vi "Header Footer Transform Header Footer [ ].vi"(7 "Header or Footer [ ]":T15, 11 "error in (no error)":errorcluster) -> (8 "Header or Footer Complete Cluster":T1, 15 "error out":errorcluster)   [LabVIEW 2019]
doc: "Version 1.0\nDeveloped by Jean-Marc Simard\nCopyright © 2010, Exaprom Inc.\nAll rights reserved.\nLicense: BSD\n\nWith iTextSharp 4.1.6 (http://itextsharp.sourceforge.net)\nunder Mozilla Public License Version 1.1\n(http://www.mozilla.org/MPL/MPL-1.1.html)"
uses:
  <userlib>/Exaprom PDF/LV Class/Header and Footer Class/VIs/Controls/Header Footer [ ] V2.ctl
  <userlib>/Exaprom PDF/LV Class/Header and Footer Class/VIs/Controls/Header Footer cluster V2.ctl
  <userlib>/Exaprom PDF/Controls/Header, Footer and Watermark Controls/Header or Footer.ctl
  <userlib>/Exaprom PDF/Controls/Header, Footer and Watermark Controls/Header Footer Type.ctl
  <userlib>/Exaprom PDF/Controls/Header, Footer and Watermark Controls/Header footer horiz alignment.ctl
  <userlib>/Exaprom PDF/Controls/Table Controls/Cell Vertical alignment.ctl
  <userlib>/Exaprom PDF/Controls/Text Controls/Line spacing.ctl
  <userlib>/Exaprom PDF/Controls/Header, Footer and Watermark Controls/Page number.ctl
  <userlib>/Exaprom PDF/Controls/Font Controls/Font complete cluster horizontal.ctl
  <userlib>/Exaprom PDF/Controls/Font Controls/Font size.ctl
  <userlib>/Exaprom PDF/Controls/Font Controls/Font color.ctl
  <userlib>/Exaprom PDF/Controls/Font Controls/Type and encoding.ctl
  <userlib>/Exaprom PDF/Controls/Text Controls/Unicode/Type and run direction.ctl
  C:/Program Files/National Instruments/LabVIEW 2019/user.lib/Exaprom PDF/DLL/itextsharp.dll
  DLL/itextsharp.dll
  <userlib>/Exaprom PDF/Controls/Header, Footer and Watermark Controls/Header Footer Line.ctl
  <userlib>/Exaprom PDF/Controls/Header, Footer and Watermark Controls/Header Footer Complete Cluster.ctl
  <userlib>/Exaprom PDF/Controls/Header, Footer and Watermark Controls/Header or Footer Position.ctl
  <userlib>/Exaprom PDF/Controls/Header, Footer and Watermark Controls/Header Footer Cluster with references.ctl
  <userlib>/Exaprom PDF/Controls/Text Controls/Text type.ctl
panel:
  # "X"
  # "Y"
  # "X"
  # "Y"
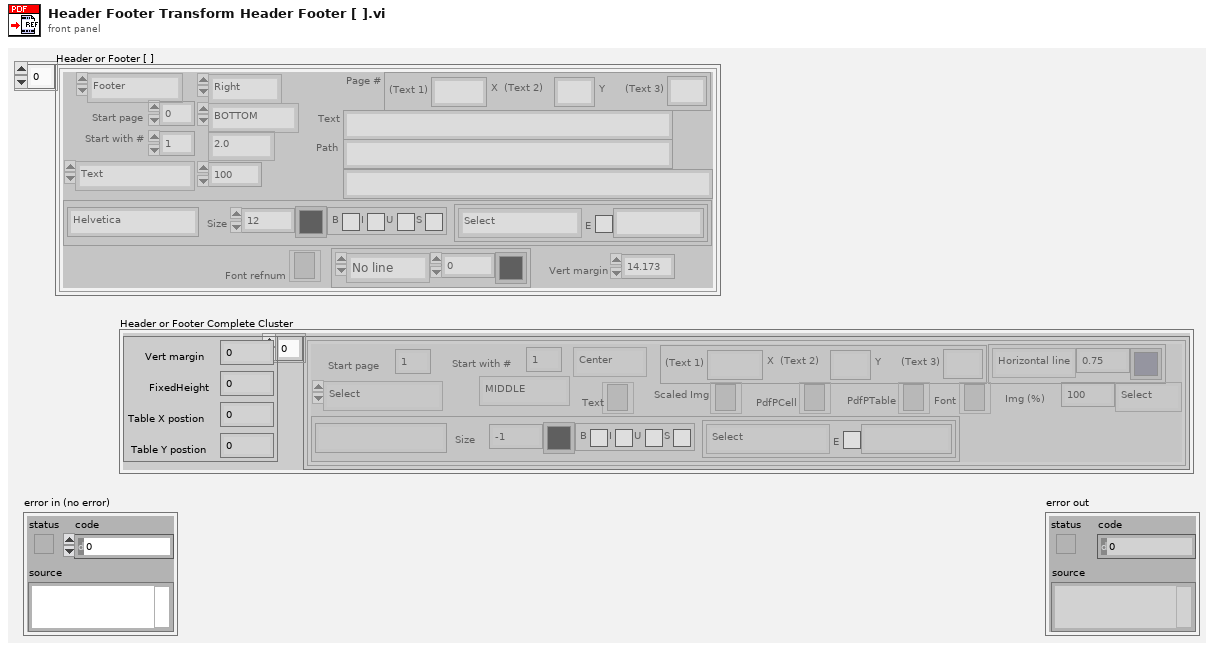
[diagram p1: front panel]
types:
  T1 = typedef "Header Footer Complete Cluster.ctl" = cluster{"Table position":T2, "Header Footer Cluster with references [ ]":T3[]}
  T2 = typedef "Header or Footer Position.ctl" = cluster{"Vert margin":dbl, "FixedHeight":dbl, "Table X postion":dbl, "Table Y postion":dbl}
  T3 = typedef "Header Footer Cluster with references.ctl" = cluster{"Start page":i32, "Type":T4, "Start with #":i32, "Alignment":T5, "Vertical Alignement":T6, "Page #":T7, "Text":refnum<k24>, "Scaled Img":refnum<k24>, "PdfPCell":refnum<k24>, "PdfPTable":refnum<k24>, "Font Cluster":T8, "Font ":refnum<k24>, "Img (%)":sgl, "Line":cluster{"Line":T13, "Thickness (points)":sgl, "Colour":T10}, "Line spacing":T14}
  T4 = typedef "Header Footer Type.ctl" = enum16{"Select", "Text", "Text + hyperlink", "Page number", "Image", "Image + hyperlink"}
  T5 = typedef "Header footer horiz alignment.ctl" = enum16{"Left", "Center", "Right"}
  T6 = typedef "Cell Vertical alignment.ctl" = enum16{"TOP", "MIDDLE", "BOTTOM"}
  T7 = typedef "Page number.ctl" = cluster{"Text 1":string, "Text 2":string, "Text 3":string}
  T8 = typedef "Font complete cluster horizontal.ctl" = cluster{"Name":string, "Size":T9, "Color":T10, "Style":cluster{"Bold":bool, "Italic":bool, "Underline":bool, "Strikeout":bool}, "Type":T11}
  T9 = typedef "Font size.ctl" = sgl
  T10 = typedef "Font color.ctl" = u32
  T11 = typedef "Type and encoding.ctl" = cluster{"Type&direction":T12, "Embedded":bool, "Encoding":string}
  T12 = typedef "Type and run direction.ctl" = enum16{"Select", "ASCII", "UTF-16", "UTF-16 (default)", "UTF-16 (LTR)", "UTF-16 (RTL)"}
  T13 = typedef "Header Footer Line.ctl" = enum16{"No line", "Horizontal line"}
  T14 = typedef "Line spacing.ctl" = enum16{"Select", "1.0", "1.5", "2.0"}
  T15 = typedef "Header Footer [ ] V2.ctl" = T16[]
  T16 = typedef "Header Footer cluster V2.ctl" = cluster{"Header or Footer":T17, "Start page":i32, "Start with #":i32, "Type":T4, "Alignment":T5, "Vertical Alignement":T6, "Line spacing":T14, "Image (%)":sgl, "Page #":T7, "Text":string, "Path":string, "Font":T8, "Font refnum":refnum<k24>, "Line":cluster{"Line":T13, "Thickness (points)":sgl, "Colour":T10}, "Vert margin":dbl, "Hyperlink":string}
  T17 = typedef "Header or Footer.ctl" = enum16{"Header", "Footer"}
  T18 = typedef "Text type.ctl" = enum16{"empty", "Text", "Hyperlink"}
  T19 = cluster{"Text type":T18, "Text":string, "Hyperlink":string}[]
  T20 = cluster{"Text type":T18, "Text":string, "Hyperlink":string}
  T21 = cluster{"Line":T13, "Thickness (points)":sgl, "Colour":T10}
  T22 = cluster{"Table position":T2, "Header Footer Cluster with references [ ]":T3[]}
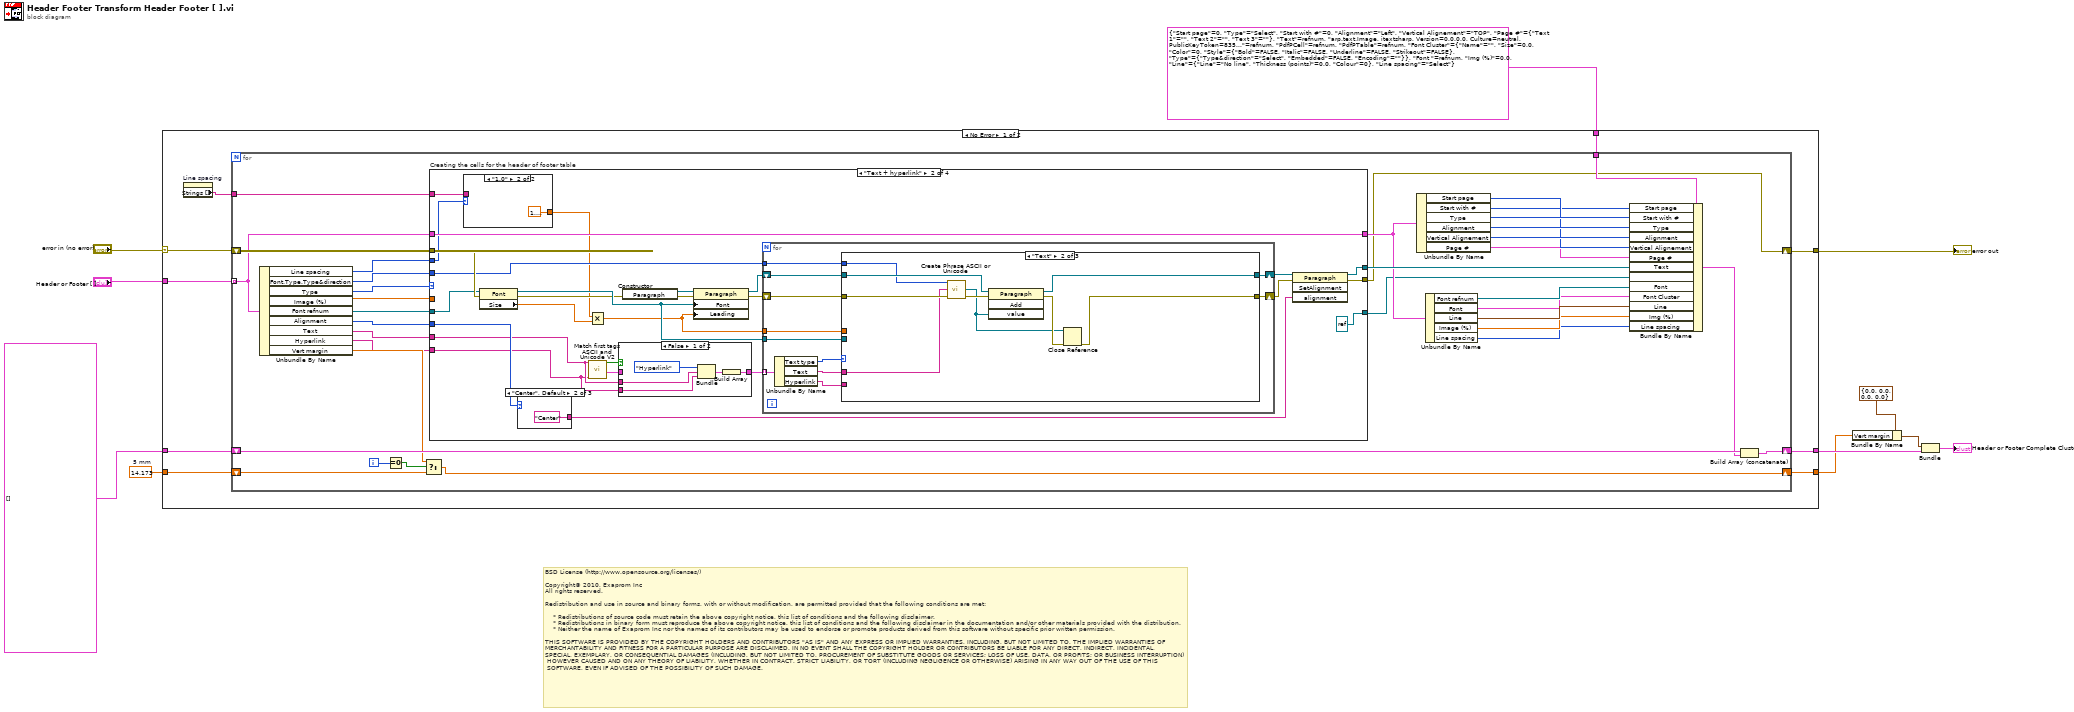
[diagram p0: block diagram]
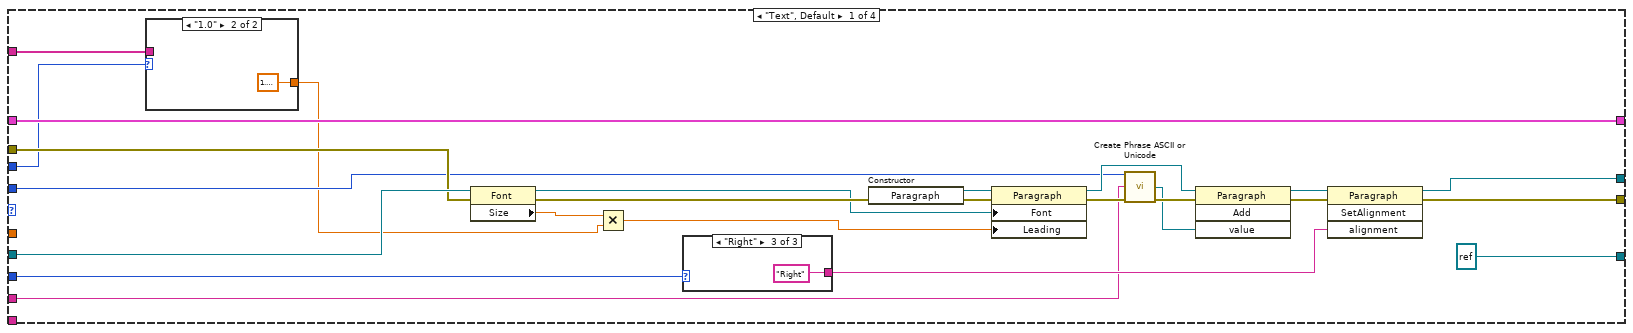
[diagram p2: hidden frame]
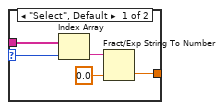
[diagram p3: hidden frame]
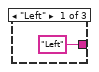
[diagram p4: hidden frame]
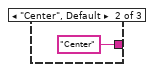
[diagram p5: hidden frame]
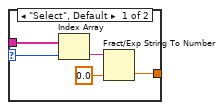
[diagram p6: hidden frame]
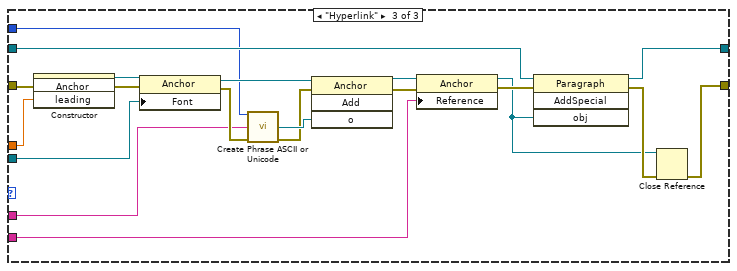
[diagram p9: hidden frame]
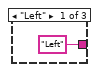
[diagram p10: hidden frame]
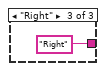
[diagram p11: hidden frame]
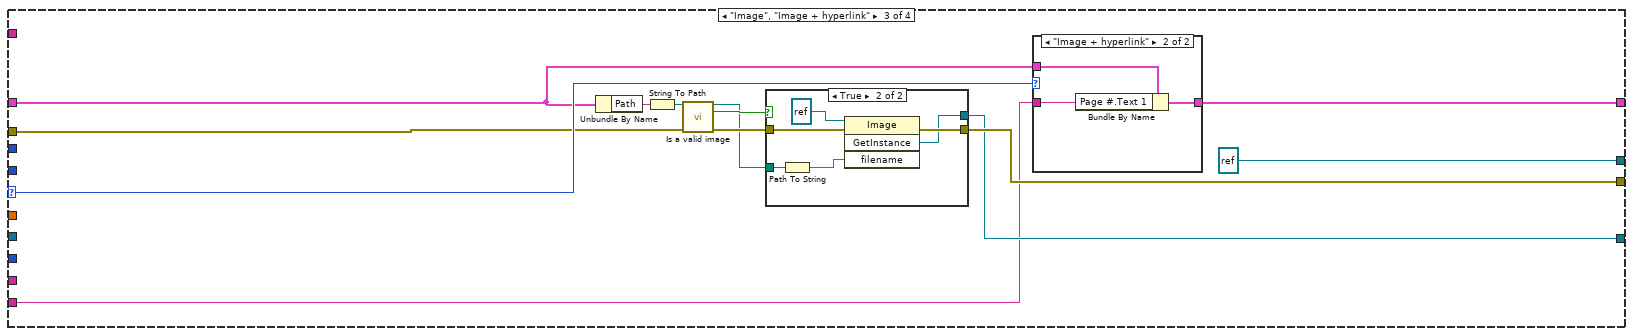
[diagram p12: hidden frame]
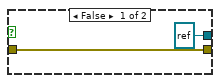
[diagram p13: hidden frame]
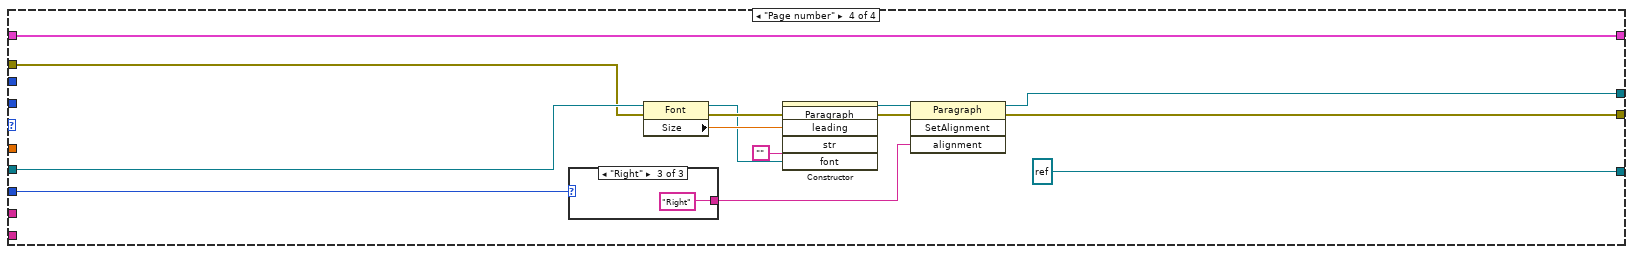
[diagram p15: hidden frame]
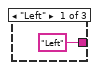
[diagram p16: hidden frame]
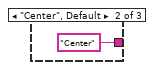
[diagram p17: hidden frame]
diagram:
  w5 = 14.173  # 5 mm
  # "BSD License (http://www.opensource.org/licenses/)\n\nCopyright© 2010, Exaprom Inc\nAll rights reserved.\n\nRedistribution and use in source and binary forms, with or without modification, are permitted provided that the following conditions are met:\n\n    * Redistributions of source code must retain the above copyright notice, this list of conditions and the following disclaimer.\n    * Redistributions in binary form must reproduce the above copyright notice, this list of conditions and the following disclaimer in the documentation and/or other materials provided with the distribution.\n    * Neither the name of Exaprom Inc nor the names of its contributors may be used to endorse or promote products derived from this software without specific prior written permission.\n\nTHIS SOFTWARE IS PROVIDED BY THE COPYRIGHT HOLDERS AND CONTRIBUTORS \"AS IS\" AND ANY EXPRESS OR IMPLIED WARRANTIES, INCLUDING, BUT NOT LIMITED TO, THE IMPLIED WARRANTIES OF \nMERCHANTABILITY AND FITNESS FOR A PARTICULAR PURPOSE ARE DISCLAIMED. IN NO EVENT SHALL THE COPYRIGHT HOLDER OR CONTRIBUTORS BE LIABLE FOR ANY DIRECT, INDIRECT, INCIDENTAL,\nSPECIAL, EXEMPLARY, OR CONSEQUENTIAL DAMAGES (INCLUDING, BUT NOT LIMITED TO, PROCUREMENT OF SUBSTITUTE GOODS OR SERVICES; LOSS OF USE, DATA, OR PROFITS; OR BUSINESS INTERRUPTION)\n HOWEVER CAUSED AND ON ANY THEORY OF LIABILITY, WHETHER IN CONTRACT, STRICT LIABILITY, OR TORT (INCLUDING NEGLIGENCE OR OTHERWISE) ARISING IN ANY WAY OUT OF THE USE OF THIS\n SOFTWARE, EVEN IF ADVISED OF THE POSSIBILITY OF SUCH DAMAGE."
  n1 = case shown="No Error" "error in (no error)" {
    selector: "error in (no error)" -> [w16 w218]
    tunnel: "Header or Footer [ ]" -> [w15 _]
    tunnel: [w20 w218] -> w11
    tunnel: T3 {"Start page"=0, "Type"=enum."Select", "Start with #"=0, "Alignment"=enum."Left", "Vertical Alignement"=enum."TOP", "Page #"={"Text 1"="", "Text 2"="", "Text 3"=""}, "Text"=refnum, "Scaled Img"=refnum, "PdfPCell"=refnum, "PdfPTable"=refnum, "Font Cluster"={"Name"="", "Size"=0.0, "Color"=0, "Style"={"Bold"=FALSE, "Italic"=FALSE, "Underline"=FALSE, "Strikeout"=FALSE}, "Type"={"Type&direction"=enum."Select", "Embedded"=FALSE, "Encoding"=""}}, "Font "=refnum, "Img (%)"=0.0, "Line"={"Line"=enum."No line", "Thickness (points)"=0.0, "Colour"=0}, "Line spacing"=enum."Select"} ("Header Footer Cluster with references") -> [w19 _]
    tunnel: T3[] [] ("Header Footer Cluster with references [ ]") -> [w18 w217]
    tunnel: [w17 w217] -> w7
    tunnel: [w14 w216] -> w2
    tunnel: w5 -> [w13 w216]
    frame No Error {
      n2 = property on="Line spacing" class="Enum (strict)"() -> ("Strings []"=w12:string[])  [unwired: 2 in, 2 out]
      n3 = for {
        tunnel: w15 -> [w41] mode=indexing
        tunnel: w19 -> [w50]
        shift-right: [w43] -> w17
        shift-left: w18 -> [w42]
        shift-right: [w36] -> w20
        shift-left: w16 -> [w39]
        shift-right: [w29] -> w14
        shift-left: w13 -> [w30]
        tunnel: w12 -> [w22]
        i -> [w32]
        n4 = Unbundle By Name(w41) -> ("Line spacing"=w23:T14, "Font.Type.Type&direction"=w27:T12, "Type"=w52:T4, "Image (%)"=w53:sgl, "Font refnum"=w55:refnum<k24>, "Alignment"=w54:T5, "Text"=w51:string, "Hyperlink"=w25:string, "Vert margin"=w26:dbl)
        n5 = Equal To 0?(x=w32) -> (x = 0?=w31:bool)
        n6 = Select(t=w26, s=w31, f=w30) -> (s? t:f=w29:dbl)
        n7 = case "Creating the cells for the header of footer table" shown="\"Text + hyperlink\"" w52 {
          selector: w52 -> [_ _ w184 _]
          tunnel: w41 -> [w75 w113 w179 w207]
          tunnel: w55 -> [w80 w98 _ w212]
          tunnel: w54 -> [w79 w116 _ w211]
          tunnel: w53 -> [_ _ _ _]
          tunnel: w51 -> [w62 w101 _ _]
          tunnel: w39 -> [w78 w99 w176 w210]
          tunnel: [w73 w111 refnum<k24> refnum ("new reference") w206] -> w44
          tunnel: [refnum<k24> refnum ("GetInstanceImage OUT") refnum<k24> refnum ("GetInstanceImage OUT") w182 refnum<k24> refnum ("GetInstanceImage OUT")] -> w38
          tunnel: [w77 w114 w185 w209] -> w36
          tunnel: [w75 w113 w183 w207] -> w40
          tunnel: w27 -> [w61 w97 _ _]
          tunnel: w25 -> [_ w100 w174 _]
          tunnel: w23 -> [w56 w91 _ _]
          tunnel: w22 -> [w59 w92 _ _]
          frame "Text", Default {
            n8 = case shown="\"1.0\"" w56 {
              selector: w56 -> [w81 _]
              tunnel: w59 -> [w83 _]
              tunnel: [w82 sgl 1.1] -> w57
              frame "Select", Default {
                n9 = Index Array(array=w83, index=w81) -> (element=w85:string)
                n10 = Fract/Exp String To Number(string=w85, default (0 dbl)=sgl 0.0 ("default (0 DBL)")) -> (number=w82:sgl)  [unwired: 3 out]
              }
              frame "1.0" {
              }
            }
            n11 = property class="Font"(reference=w80, error in=w78) -> (reference out=w69:refnum<k24>, error out=w72:errorcluster, "Size"=w68:sgl)
            n12 = Multiply(x=w68, y=w57) -> (x*y=w58:sgl)
            n13 = case shown="\"Right\"" w79 {
              tunnel: ["Left" "Center" "Right"] -> w74
              frame "Left" {
              }
              frame "Center", Default {
              }
              frame "Right" {
              }
            }
            n14 = constructor class="Paragraph"(error in=w72) -> (reference out=w70:refnum<k24>, error out=w71:errorcluster)  [unwired: 2 in, 1 out]
            n15 = property class="Paragraph"(reference=w70, error in=w71, "Font"=w69, "Leading"=w58) -> (reference out=w65:refnum<k24>, error out=w64:errorcluster)
            n16 = call <userlib>:"Create Phrase ASCII or Unicode.vi"("Character type"=w61, "Text"=w62, "error in (no error)"=w64) -> ("Phrase refnum"=w60:refnum<k24>, "error out"=w63:errorcluster)  [unwired: 10 in, 1 out]
            n17 = invoke class="Paragraph" method="Add"(reference=w65, error in=w63, "value"=w60) -> (reference out=w67:refnum<k24>, error out=w66:errorcluster)  [unwired: 1 in, 2 out]
            n18 = invoke class="Paragraph" method="SetAlignment"(reference=w67, error in=w66, "alignment"=w74) -> (reference out=w73:refnum<k24>, error out=w77:errorcluster)  [unwired: 1 in, 2 out]
          }
          frame "Text + hyperlink" {
            n19 = case shown="\"1.0\"" w91 {
              selector: w91 -> [w117 _]
              tunnel: w92 -> [w119 _]
              tunnel: [w118 sgl 1.1] -> w90
              frame "Select", Default {
                n20 = Index Array(array=w119, index=w117) -> (element=w121:string)
                n21 = Fract/Exp String To Number(string=w121, default (0 dbl)=sgl 0.0 ("default (0 DBL)")) -> (number=w118:sgl)  [unwired: 3 out]
              }
              frame "1.0" {
              }
            }
            n22 = property class="Font"(reference=w98, error in=w99) -> (reference out=w110:refnum<k24>, error out=w105:errorcluster, "Size"=w109:sgl)
            n23 = case shown="\"Center\", Default" w116 {
              tunnel: ["Left" "Center" "Right"] -> w112
              frame "Left" {
              }
              frame "Center", Default {
              }
              frame "Right" {
              }
            }
            n24 = Multiply(x=w90, y=w109) -> (x*y=w93:sgl)
            n25 = call <userlib>:"Match first tags ASCII and Unicode V2.vi"("Hyperlink"=w100, "Text"=w101) -> ("Array"=w108:T19, "Find tag ?"=w106:bool)  [unwired: 3 in, 5 out]
            n26 = case shown="False" w106 {
              tunnel: [w123 w128] -> w107
              tunnel: w108 -> [_ w128]
              tunnel: w101 -> [w125 _]
              tunnel: w100 -> [w126 _]
              frame False {
                n27 = Bundle("Text type"=Text_type."Hyperlink", "Text"=w125, "Hyperlink"=w126) -> (w127:T20)  [unwired: 1 in]
                n28 = Build Array(w127) -> (w123:T19)
              }
              frame True {
              }
            }
            n29 = constructor class="Paragraph"(error in=w105) -> (reference out=w103:refnum<k24>, error out=w104:errorcluster)  [unwired: 2 in, 1 out]
            n30 = property class="Paragraph"(reference=w103, error in=w104, "Font"=w110, "Leading"=w93) -> (reference out=w94:refnum<k24>, error out=w102:errorcluster)
            n31 = for {
              shift-right: [w137] -> w95
              shift-left: w94 -> [w138]
              shift-right: [w136] -> w96
              shift-left: w102 -> [w139]
              tunnel: w107 -> [w135] mode=indexing
              tunnel: w93 -> [w131]
              tunnel: w110 -> [w130]
              tunnel: w97 -> [w129]
              n32 = Unbundle By Name(w135) -> ("Text type"=w134:T18, "Text"=w133:string, "Hyperlink"=w132:string)
              n33 = case shown="\"Text\"" w134 {
                tunnel: w139 -> [w141 w149 w164]
                tunnel: w138 -> [w140 w148 w159]
                tunnel: [w140 w147 w160] -> w137
                tunnel: [w141 w144 w155] -> w136
                tunnel: w133 -> [_ w146 w158]
                tunnel: w132 -> [_ _ w157]
                tunnel: w131 -> [_ _ w153]
                tunnel: w130 -> [_ _ w152]
                tunnel: w129 -> [_ w142 w151]
                frame "empty", Default {
                }
                frame "Text" {
                  n34 = call <userlib>:"Create Phrase ASCII or Unicode.vi"("Character type"=w142, "Text"=w146, "error in (no error)"=w149) -> ("Phrase refnum"=w143:refnum<k24>, "error out"=w150:errorcluster)  [unwired: 10 in, 1 out]
                  n35 = invoke class="Paragraph" method="Add"(reference=w148, error in=w150, "value"=w143) -> (reference out=w147:refnum<k24>, error out=w145:errorcluster)  [unwired: 1 in, 2 out]
                  n36 = Close Reference(reference=w143, error in (no error)=w145) -> (error out=w144:errorcluster)
                }
                frame "Hyperlink" {
                  n37 = constructor class="Anchor"(error in=w164, "leading"=w153) -> (reference out=w170:refnum<k24>, error out=w169:errorcluster)  [unwired: 2 in, 2 out]
                  n38 = property class="Anchor"(reference=w170, error in=w169, "Font"=w152) -> (reference out=w168:refnum<k24>, error out=w163:errorcluster)
                  n39 = call <userlib>:"Create Phrase ASCII or Unicode.vi"("Character type"=w151, "Text"=w158, "error in (no error)"=w163) -> ("Phrase refnum"=w165:refnum<k24>, "error out"=w162:errorcluster)  [unwired: 10 in, 1 out]
                  n40 = invoke class="Anchor" method="Add"(reference=w168, error in=w162, "o"=w165) -> (reference out=w166:refnum<k24>, error out=w167:errorcluster)  [unwired: 1 in, 2 out]
                  n41 = property class="Anchor"(reference=w166, error in=w167, "Reference"=w157) -> (reference out=w154:refnum<k24>, error out=w161:errorcluster)
                  n42 = invoke class="Paragraph" method="AddSpecial"(reference=w159, error in=w161, "obj"=w154) -> (reference out=w160:refnum<k24>, error out=w156:errorcluster)  [unwired: 1 in, 2 out]
                  n43 = Close Reference(reference=w154, error in (no error)=w156) -> (error out=w155:errorcluster)
                }
              }
            }
            n44 = invoke class="Paragraph" method="SetAlignment"(reference=w95, error in=w96, "alignment"=w112) -> (reference out=w111:refnum<k24>, error out=w114:errorcluster)  [unwired: 1 in, 2 out]
          }
          frame "Image", "Image + hyperlink" {
            n45 = Unbundle By Name(w179) -> ("Path"=w180:string)
            n46 = String To Path(string=w180) -> (path=w181:path)
            n47 = call <userlib>:"Is a valid image.vi"("Image path"=w181, "error in (no error)"=w176) -> ("dup path"=w175:path, "Valid Image?"=w178:bool, "error out"=w177:errorcluster)  [unwired: 11 out]
            n48 = case shown="True" w178 {
              tunnel: w175 -> [_ w193]
              tunnel: [w188 w192] -> w185
              tunnel: [refnum<k24> refnum ("GetInstance") w191] -> w182
              tunnel: w177 -> [w188 w190]
              frame False {
              }
              frame True {
                n49 = Path To String(path=w193) -> (string=w189:string)
                n50 = invoke class="Image" method="GetInstance"(reference=refnum<k24> refnum ("image"), error in=w190, "filename"=w189) -> (error out=w192:errorcluster, "GetInstance"=w191:refnum<k24>)  [unwired: 1 in, 2 out]
              }
            }
            n51 = case shown="\"Image + hyperlink\"" w184 {
              tunnel: [w195 w197] -> w183
              tunnel: w179 -> [w195 w198]
              tunnel: w174 -> [_ w196]
              frame "Select", Default {
              }
              frame "Image + hyperlink" {
                n52 = Bundle By Name(cluster=w198, "Page #.Text 1"=w196) -> (w197:T16)
              }
            }
          }
          frame "Page number" {
            n53 = case shown="\"Right\"" w211 {
              tunnel: ["Left" "Center" "Right"] -> w203
              frame "Left" {
              }
              frame "Center", Default {
              }
              frame "Right" {
              }
            }
            n54 = property class="Font"(reference=w212, error in=w210) -> (reference out=w200:refnum<k24>, error out=w202:errorcluster, "Size"=w201:sgl)
            n55 = constructor class="Paragraph"(error in=w202, "leading"=w201, "str"="", "font"=w200) -> (reference out=w204:refnum<k24>, error out=w199:errorcluster)  [unwired: 2 in, 4 out]
            n56 = invoke class="Paragraph" method="SetAlignment"(reference=w204, error in=w199, "alignment"=w203) -> (reference out=w206:refnum<k24>, error out=w209:errorcluster)  [unwired: 1 in, 2 out]
          }
        }
        n57 = Unbundle By Name(w40) -> ("Start page"=w28:i32, "Start with #"=w49:i32, "Type"=w48:T4, "Alignment"=w47:T5, "Vertical Alignement"=w46:T6, "Page #"=w45:T7)
        n58 = Unbundle By Name(w40) -> ("Font refnum"=w34:refnum<k24>, "Font"=w21:T8, "Line"=w35:T21, "Image (%)"=w33:sgl, "Line spacing"=w24:T14)
        n59 = Bundle By Name(cluster=w50, "Start page"=w28, "Start with #"=w49, "Type"=w48, "Alignment"=w47, "Vertical Alignement"=w46, "Page #"=w45, "Text"=w44, "Scaled Img"=w38, "Font"=w34, "Font Cluster"=w21, "Line"=w35, "Img (%)"=w33, "Line spacing"=w24) -> (w37:T3)
        n60 = Build Array (concatenate)(w42, w37) -> (w43:T3[])
      }
    }
    frame Error {
    }
  }
  "error out" <- w11
  n61 = Bundle By Name(cluster=T2 {"Vert margin"=0.0, "FixedHeight"=0.0, "Table X postion"=0.0, "Table Y postion"=0.0} ("Table position"), "Vert margin"=w2) -> (w3:T2)
  n62 = Bundle("Table position"=w3, "Header Footer Cluster with references [ ]"=w7) -> (→"Header or Footer Complete Cluster":T22)  [unwired: 1 out]
